vi "OutletPostRequest.vi"(1 "SwitchInput":i32, 2 "NameInput":string) -> ()   [LabVIEW 2014]
uses:
  <vilib>/httpClient/POSTBuffer.vi
  <vilib>/httpClient/LabVIEWHTTPClient.lvlib
panel:
  in  "?":cluster{"name":string, "switch":i32}
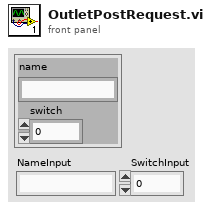
[diagram p1: front panel]
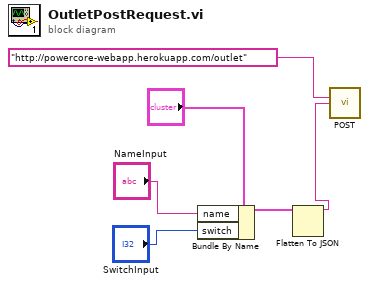
[diagram p0: block diagram]
diagram:
  n1 = Bundle By Name(cluster="?", "name"="NameInput", "switch"="SwitchInput") -> (w3:cluster{"name":string, "switch":i32})
  n2 = Flatten To JSON(anything=w3) -> (JSON string=w5:string)  [unwired: 2 in, 1 out]
  n3 = call-poly <vilib>:"POST.vi"("url"="http://powercore-webapp.herokuapp.com/outlet", "buffer"=w5) -> ()  [unwired: 10 in, 4 out]
